vi "DAQX mod 1SDI v02.vi"(0 "resource names":T3={"resource 1"="PXI1Slot2", "resource 2"="PXI1Slot2"}, 1 "close (T)":bool=TRUE, 2 "Record Data":bool, 3 "numSamples":i32=-1, 4 "max time (s)":dbl=10.0 caption="max time", 5 "min sample rate":dbl=100000000.0, 6 "File location":path, 7 "error in":errorcluster, 8 "reference position":dbl=50.0, 9 "Additional text":string, 10 "Type of measurement":T4, 11 "Name root":string, 12 "Monitor On":bool, 13 "channel parameters":T6(array[cluster])=[{"channel name"="0", "input impedance"=0, "maximum input frequency"=30000000.0, "vertical coupling"=1, "probe attenuation"=1.0, "vertical range"=2.0, "vertical offset"=0.0, "channel enabled"=TRUE}, {"channel name"="1", "input impedance"=0, "maximum input frequency"=30000000.0, "vertical coupling"=1, "probe attenuation"=1.0, "vertical range"=2.0, "vertical offset"=0.0, "channel enabled"=TRUE}] {"input impedance" items=["1 mega ohm"=0, "50 ohms"=2]; "vertical coupling" items=["AC", "DC", "Ground"]}, 15 "reset sn":bool) -> (16 "wfm out 1":waveform(dbl)[](array[waveform]), 18 "wfm out 2":waveform(dbl)[](array[waveform]), 19 "file saved":path, 22 "Parameters values file":string, 24 "actualSamples 2":i32, 26 "actualSamples 3":i32, 27 "error out 2":errorcluster caption="error out final")   [LabVIEW 2013]
doc: "Configures and acquires data from an NI-SCOPE high-speed digitizer.\n--------------------\n\nThis Express VI is configured as follows:\n\nDevice: PXI1Slot2 (PXI-5122)\nSample Rate (S/s): 100M\nRecord length: 2k\nAcquisition Mode: N Samples\nChannel 0\n - Range (V): 2\n - Offset (V): 0\n - Probe attenuation: 1\n - Coupling: \n - Input impedence: 1 \n - Bandwidth (Hz): 0\nChannel 1\n - Range (V): 2\n - Offset (V): 0\n - Probe attenuation: 1\n - Coupling: \n - Input impedence: 1 \n - Bandwidth (Hz): 0\nImmediate"
uses:
  <instrlib>/niScope/Controls/niScope vertical coupling.ctl
  Strict Type Defs/type_meas_enum.ctl
  <instrlib>/niScope/Controls/niScope timestamp type.ctl
  <instrlib>/niScope/Controls/niScope clock sync pulse source.ctl
  <instrlib>/niScope/Controls/niScope trigger source digital.ctl
  <instrlib>/niScope/Controls/niScope export destinations.ctl
  <instrlib>/niScope/Controls/niScope exportable signals.ctl
  <instrlib>/niScope/Acquire/Fetch/niScope Multi Fetch Binary 16.vi
  <instrlib>/niScope/Configure/Trigger/niScope Configure Trigger Digital.vi
  <instrlib>/niScope/Configure/Trigger/niScope Configure Trigger Immediate.vi
  shotnoise.vi
  <instrlib>/niScope/Acquire/Fetch/niScope Multi Fetch WDT.vi
panel:
  out "error out 1":errorcluster caption="error out final"
  out "actualSamples 1":i32
  out "actualSamples 0":i32
  out "Chan 1 params":T1
  out "Chan 0 params":T1
  out "actual sample rate":T2
  out "Chan 3 params":T1
  out "Chan 2 params":T1
  out "file location into parameter files":path
  out "size(s)":i32
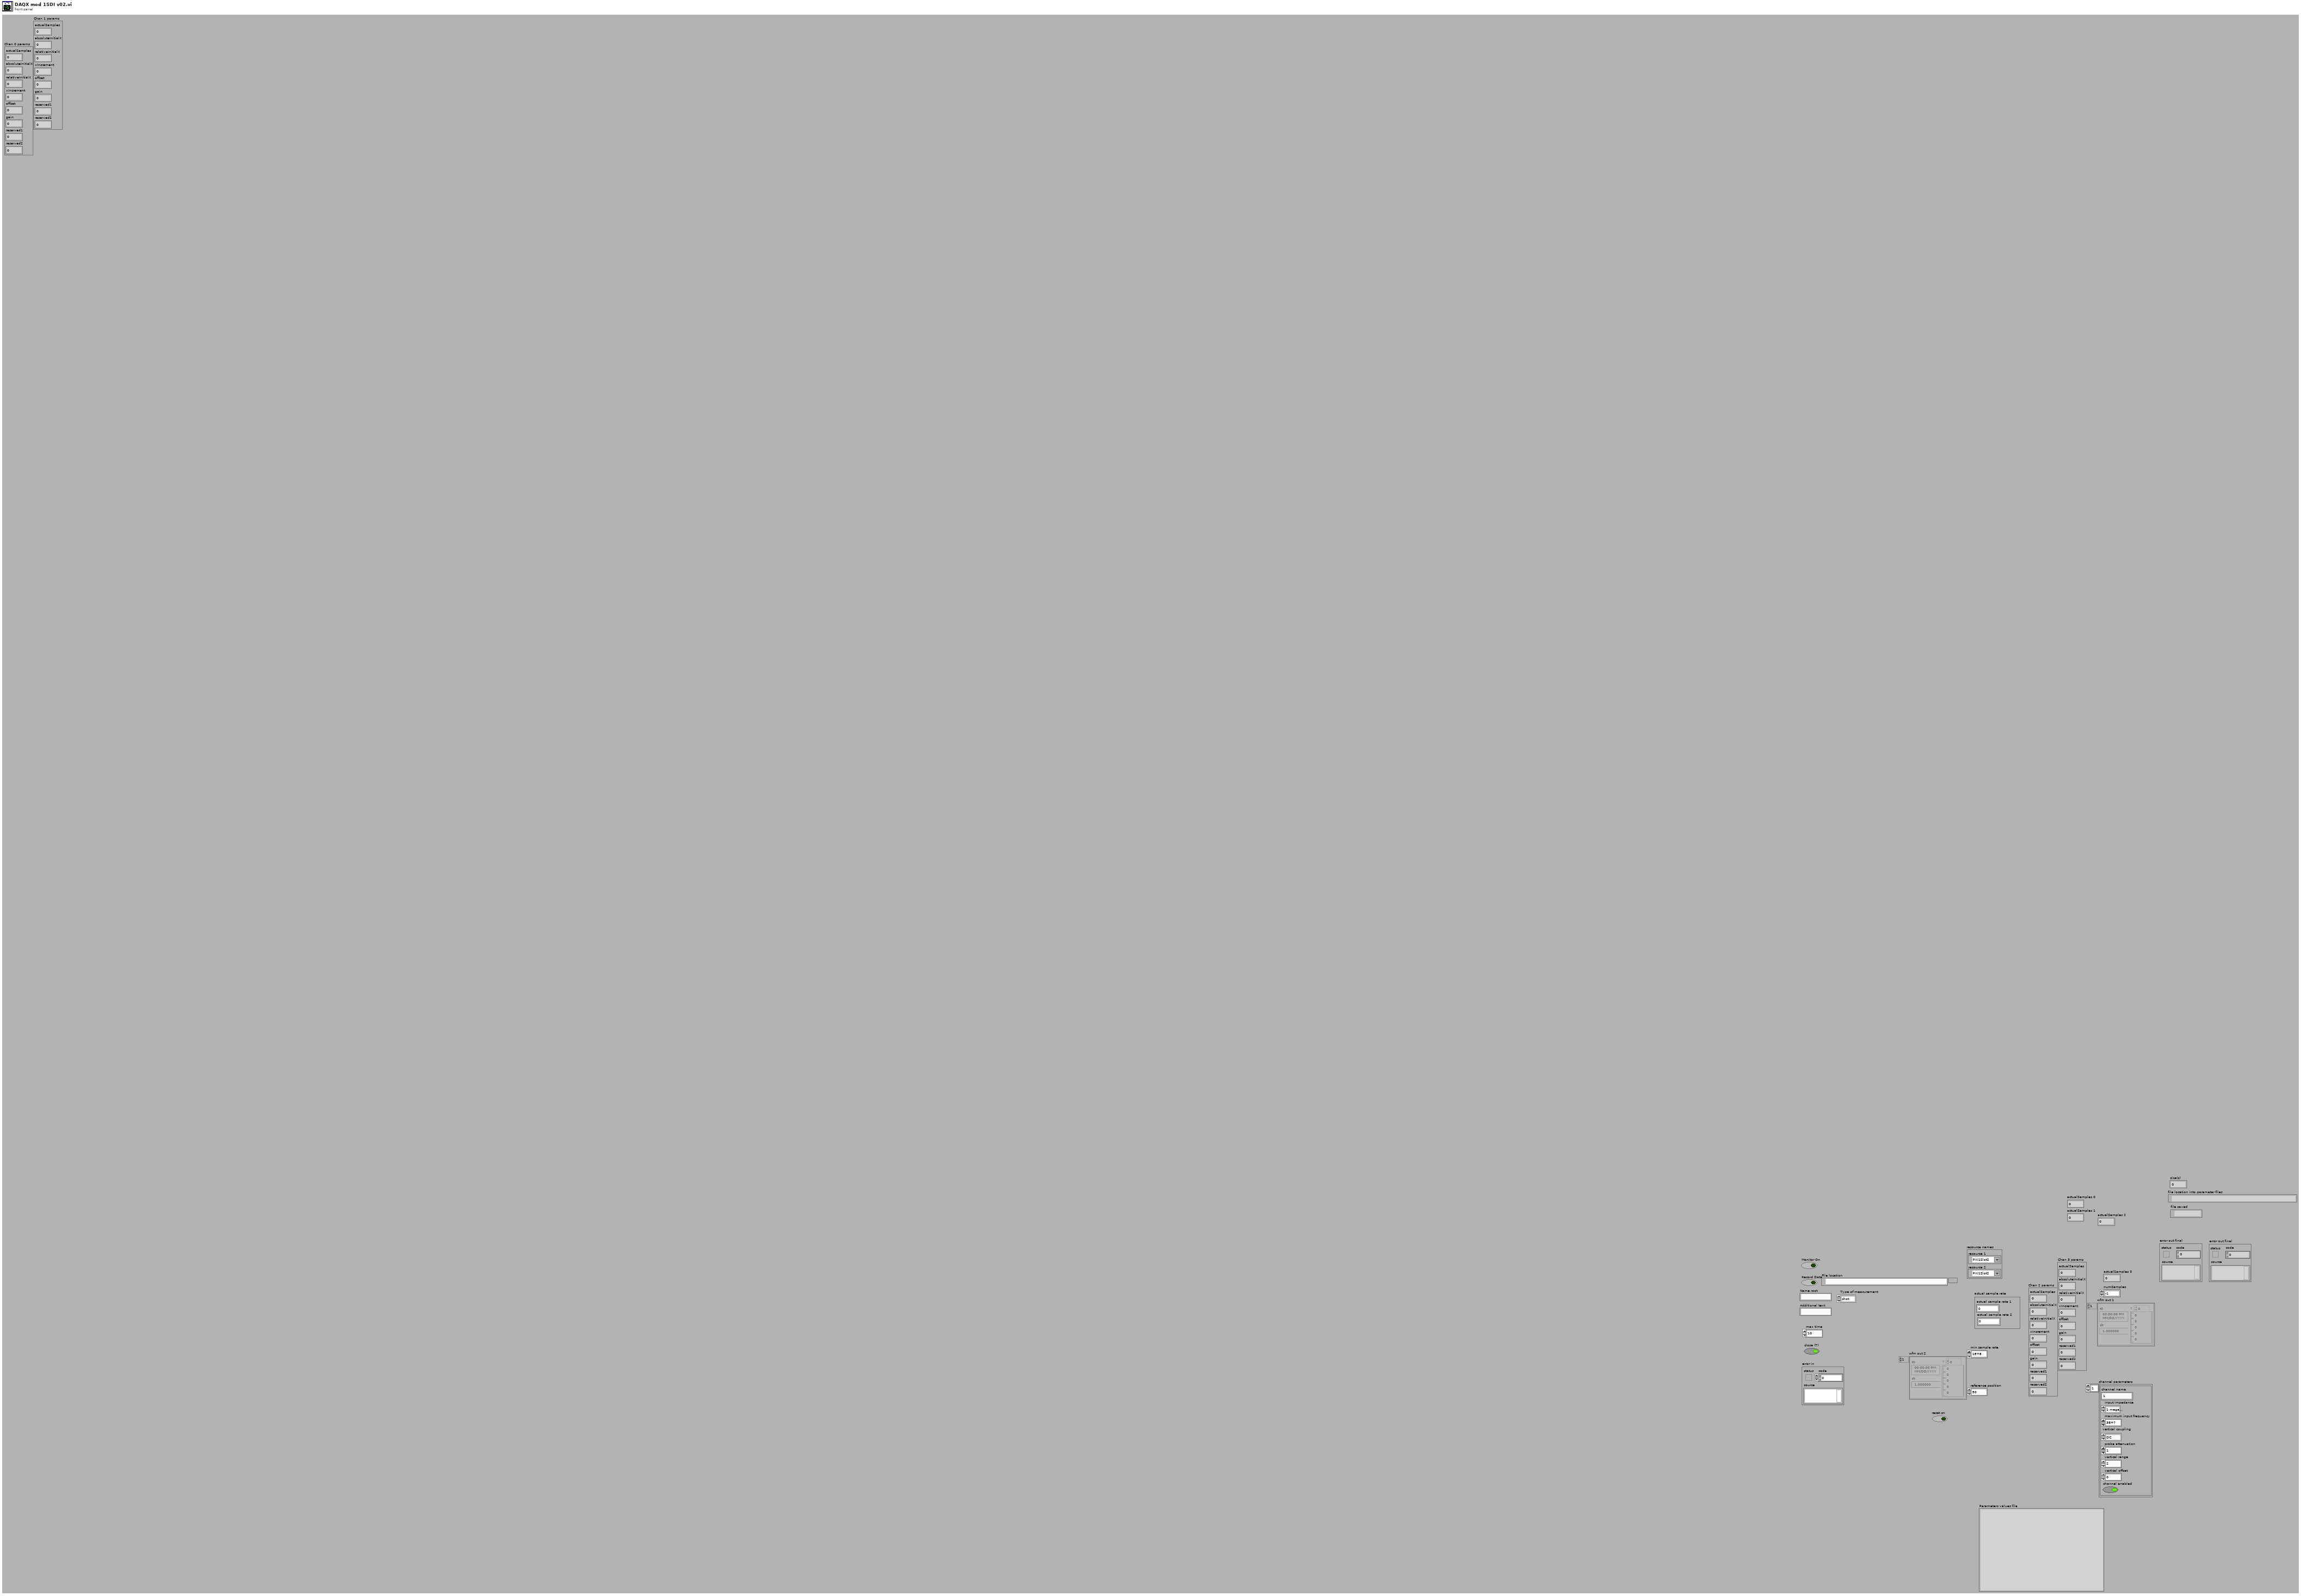
[diagram p1: front panel]
types:
  T1 = cluster{"actualSamples":i32, "absoluteInitialX":dbl, "relativeInitialX":dbl, "xIncrement":dbl, "offset":dbl, "gain":dbl, "reserved1":dbl, "reserved2":dbl}
  T2 = cluster{"actual sample rate":dbl, "actual sample rate 2":dbl}
  T3 = cluster{"resource 1":refnum<k15>, "resource 2":refnum<k15>}
  T4 = typedef "type_meas_enum.ctl" = enum16{"shot", "x", "p", "electronic"}
  T5 = typedef "niScope vertical coupling.ctl" = i32
  T6 = cluster{"channel name":string, "input impedance":u32, "maximum input frequency":dbl, "vertical coupling":T5, "probe attenuation":dbl, "vertical range":dbl, "vertical offset":dbl, "channel enabled":bool}[]
  T7 = typedef "niScope timestamp type.ctl" = i32
  T8 = typedef "niScope export destinations.ctl" = string
  T9 = typedef "niScope trigger source digital.ctl" = string
  T10 = typedef "niScope exportable signals.ctl" = u16
  T11 = typedef "niScope clock sync pulse source.ctl" = u16
  T12 = cluster{"actual sample rate":dbl, "actual sample rate":dbl}
  T13 = cluster{"actualSamples":i32, "absoluteInitialX":dbl, "relativeInitialX":dbl, "xIncrement":dbl, "offset":dbl, "gain":dbl, "reserved1":dbl, "reserved2":dbl}[]
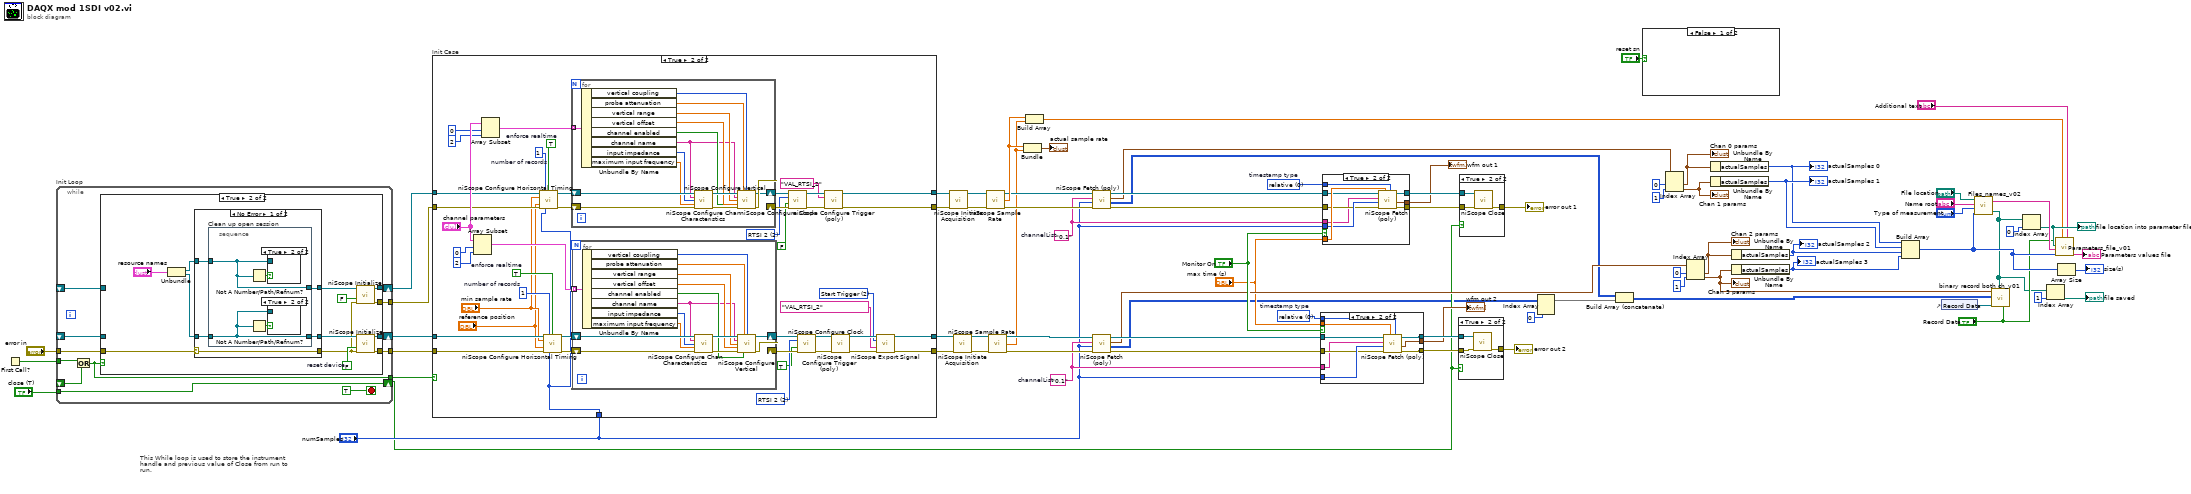
[diagram p0: block diagram]
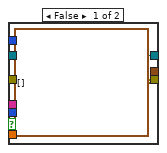
[diagram p3: hidden frame]
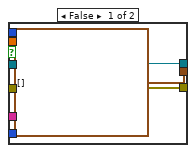
[diagram p4: hidden frame]
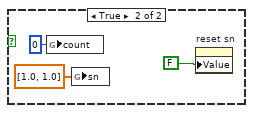
[diagram p5: hidden frame]
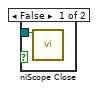
[diagram p7: hidden frame]
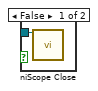
[diagram p8: hidden frame]
diagram:
  w28 = T7 0 items=["relative", "absolute"]  # timestamp type
  w31 = "0,1"  # channelList
  w44 = "0,1"  # channelList
  w78 = T7 0 items=["relative", "absolute"]  # timestamp type
  # "This While loop is used to store the instrument handle and previous value of Close from run to run."
  n1 = First Call?() -> (First Call?: T/F=w77:bool)
  n2 = while "Init Loop" {
    tunnel: w77 -> [w91]
    shift-right: [w90] -> w22
    shift-left: _ -> [w87]
    tunnel: "close (T)" -> [w90]
    shift-right: [w89] -> w76
    shift-left: _ -> [w88]
    tunnel: [w85] -> w75
    tunnel: "error in" -> [w84]
    tunnel: [w80] -> w74
    shift-right: [w83] -> w39
    shift-left: _ -> [w82]
    tunnel: [w81] -> w40
    stop <- TRUE ("stopInit") stop-if-true
    n3 = Or(x=w91, y=w87) -> (x .or. y?=w80:bool)
    n4 = case "Select_Init" shown="True" w80 {
      tunnel: [w94 w105] -> w89
      tunnel: w88 -> [w94 _]
      tunnel: [w92 w104] -> w85
      tunnel: w84 -> [w92 w103]
      tunnel: [w93 w98] -> w83
      tunnel: w82 -> [w93 _]
      tunnel: [w92 w95] -> w81
      frame False {
      }
      frame True {
        w106 = FALSE  # reset device
        n5 = Unbundle("resource names") -> ("resource 1"=w100:refnum<k15>, "resource 2"=w101:refnum<k15>)
        n6 = case shown="No Error" w103 {
          selector: w103 -> [w110 w120]
          tunnel: [w112 w121] -> w107
          tunnel: w101 -> [w111 w121]
          tunnel: [w110 w120] -> w97
          tunnel: w100 -> [w109 w119]
          tunnel: [w108 w119] -> w99
          frame No Error {
            n7 = stacked-sequence "Clean up open session" {
              tunnel: w111 -> [w115]
              tunnel: [w115] -> w112
              tunnel: w109 -> [w113]
              tunnel: [w113] -> w108
              frame #0 {
                n8 = Not A Number/Path/Refnum?(number/path/refnum=w113) -> (NaN/Path/Refnum?=w114:bool)
                n9 = Not A Number/Path/Refnum?(number/path/refnum=w115) -> (NaN/Path/Refnum?=w116:bool)
                n10 = case shown="True" w114 {
                  tunnel: w113 -> [w117 _]
                  frame False {
                    n11 = call <instrlib>:"niScope Close.vi"("instrument handle"=w117) -> ()  [unwired: 1 in, 14 out]
                  }
                  frame True {
                  }
                }
                n12 = case shown="True" w116 {
                  tunnel: w115 -> [w118 _]
                  frame False {
                    n13 = call <instrlib>:"niScope Close.vi"("instrument handle"=w118) -> ()  [unwired: 1 in, 14 out]
                  }
                  frame True {
                  }
                }
              }
            }
          }
          frame Error {
          }
        }
        n14 = call <instrlib>:"niScope Initialize.vi"("resource name"=w99, "reset device"=FALSE, "error in"=w97) -> ("instrument handle"=w98:refnum<k15>, "error out"=w95:errorcluster)  [unwired: 2 in, 9 out]
        n15 = call <instrlib>:"niScope Initialize.vi"("resource name"=w107, "reset device"=w106, "error in"=w97) -> ("instrument handle"=w105:refnum<k15>, "error out"=w104:errorcluster)  [unwired: 2 in, 9 out]
      }
    }
  }
  n16 = case "Init Case" shown="True" w74 {
    tunnel: w75 -> [w124 w163]
    tunnel: [w124 w132] -> w7
    tunnel: [w125 w133] -> w8
    tunnel: w76 -> [w125 w164]
    tunnel: "numSamples" -> [_ w128]
    tunnel: w40 -> [w122 w153]
    tunnel: w39 -> [w123 w152]
    tunnel: [w123 w127] -> w6
    tunnel: [w122 w126] -> w5
    frame False {
    }
    frame True {
      w131 = T10 2 items=["None"=0, "Start Trigger"=2, "Advance Trigger"=5, "Reference Trigger"=1, "End of Record Event"=4, "End of Acquisition Event"=3, "Ready for Start Event"=7, "Ready for Advance Event"=6, "Ready for Reference Event"=10, "Reference Clock"=100, "Sample Clock"=101, "5 Volt Power"=13] ("signal")
      w144 = T11 2 items=["RTSI 0", "RTSI 1", "RTSI 2", "RTSI 3", "RTSI 4", "RTSI 5", "RTSI 6", "PFI 1", "PFI 2", "Internal"] ("clock sync pulse source")
      w145 = T11 2 items=["RTSI 0", "RTSI 1", "RTSI 2", "RTSI 3", "RTSI 4", "RTSI 5", "RTSI 6", "PFI 1", "PFI 2", "Internal"] ("clock sync pulse source")
      w151 = 1  # number of records
      w150 = TRUE  # enforce realtime
      w167 = 1  # number of records
      w168 = TRUE  # enforce realtime
      n17 = Array Subset(array="channel parameters", index=0, length=2) -> (w160:T6)
      n18 = Array Subset(array="channel parameters", index=0, length=2) -> (w158:T6)
      n19 = call <instrlib>:"niScope Configure Horizontal Timing.vi"("instrument handle"=w152, "number of records"=w151, "enforce realtime"=w150, "min sample rate"="min sample rate", "reference position"="reference position", "error in"=w153, "min record length"=w128) -> ("instrument handle out"=w155:refnum<k15>, "error out"=w154:errorcluster)  [unwired: 7 out]
      n20 = call <instrlib>:"niScope Configure Horizontal Timing.vi"("instrument handle"=w164, "number of records"=w167, "enforce realtime"=w168, "min sample rate"="min sample rate", "reference position"="reference position", "error in"=w163, "min record length"=w128) -> ("instrument handle out"=w165:refnum<k15>, "error out"=w166:errorcluster)  [unwired: 7 out]
      n21 = for {
        shift-right: [w171] -> w148
        shift-left: w154 -> [w183]
        shift-right: [w170] -> w149
        shift-left: w155 -> [w182]
        tunnel: w158 -> [w179] mode=indexing
        n22 = Unbundle By Name(w179) -> ("vertical coupling"=w176:T5, "probe attenuation"=w175:dbl, "vertical range"=w174:dbl, "vertical offset"=w173:dbl, "channel enabled"=w172:bool, "channel name"=w169:string, "input impedance"=w177:u32, "maximum input frequency"=w178:dbl)
        n23 = call <instrlib>:"niScope Configure Chan Characteristics.vi"("instrument handle"=w182, "channels"=w169, "input impedance"=w177, "maximum input frequency"=w178, "error in"=w183) -> ("instrument handle out"=w181:refnum<k15>, "error out"=w180:errorcluster)  [unwired: 9 out]
        n24 = call <instrlib>:"niScope Configure Vertical.vi"("instrument handle"=w181, "probe attenuation"=w175, "vertical coupling"=w176, "channels"=w169, "vertical range"=w174, "vertical offset"=w173, "error in"=w180, "channel enabled"=w172) -> ("instrument handle out"=w170:refnum<k15>, "error out"=w171:errorcluster)  [unwired: 6 out]
      }
      n25 = for {
        shift-right: [w186] -> w146
        shift-left: w166 -> [w198]
        shift-right: [w185] -> w147
        shift-left: w165 -> [w197]
        tunnel: w160 -> [w194] mode=indexing
        n26 = Unbundle By Name(w194) -> ("vertical coupling"=w191:T5, "probe attenuation"=w190:dbl, "vertical range"=w189:dbl, "vertical offset"=w188:dbl, "channel enabled"=w187:bool, "channel name"=w184:string, "input impedance"=w192:u32, "maximum input frequency"=w193:dbl)
        n27 = call <instrlib>:"niScope Configure Chan Characteristics.vi"("instrument handle"=w197, "channels"=w184, "input impedance"=w192, "maximum input frequency"=w193, "error in"=w198) -> ("instrument handle out"=w196:refnum<k15>, "error out"=w195:errorcluster)  [unwired: 9 out]
        n28 = call <instrlib>:"niScope Configure Vertical.vi"("instrument handle"=w196, "probe attenuation"=w190, "vertical coupling"=w191, "channels"=w184, "vertical range"=w189, "vertical offset"=w188, "error in"=w195, "channel enabled"=w187) -> ("instrument handle out"=w185:refnum<k15>, "error out"=w186:errorcluster)  [unwired: 6 out]
      }
      n29 = call <instrlib>:"niScope Configure Clock.vi"("instrument handle"=w149, "clock sync pulse source"=w144, "master enabled"=FALSE, "error in"=w148) -> ("instrument handle out"=w136:refnum<k15>, "error out"=w137:errorcluster)  [unwired: 10 in]
      n30 = call <instrlib>:"niScope Configure Clock.vi"("instrument handle"=w147, "clock sync pulse source"=w145, "master enabled"=TRUE, "error in"=w146) -> ("instrument handle out"=w141:refnum<k15>, "error out"=w140:errorcluster)  [unwired: 10 in]
      n31 = call-poly <instrlib>:"niScope Configure Trigger (poly).vi"("instrument handle"=w136, "trigger source"=T9 "VAL_RTSI_2", "error in"=w137) -> ("instrument handle out"=w127:refnum<k15>, "error out"=w126:errorcluster)  [unwired: 3 in, 8 out]
      n32 = call-poly <instrlib>:"niScope Configure Trigger (poly).vi"("instrument handle"=w141, "error in"=w140) -> ("instrument handle out"=w139:refnum<k15>, "error out"=w138:errorcluster)  [unwired: 12 out]
      n33 = call <instrlib>:"niScope Export Signal.vi"("instrument handle"=w139, "signal"=w131, "output terminal"=T8 "VAL_RTSI_2", "error in"=w138) -> ("instrument handle out"=w133:refnum<k15>, "error out"=w132:errorcluster)  [unwired: 10 in]
    }
  }
  n34 = call <instrlib>:"niScope Initiate Acquisition.vi"("instrument handle"=w6, "error in"=w5) -> ("instrument handle out"=w2:refnum<k15>, "error out"=w1:errorcluster)  [unwired: 12 out]
  n35 = call <instrlib>:"niScope Initiate Acquisition.vi"("instrument handle"=w8, "error in"=w7) -> ("instrument handle out"=w4:refnum<k15>, "error out"=w3:errorcluster)  [unwired: 12 out]
  n36 = call <instrlib>:"niScope Sample Rate.vi"("instrument handle"=w2, "error in"=w1) -> ("instrument handle out"=w36:refnum<k15>, "actual sample rate"=w37:dbl, "error out"=w35:errorcluster)  [unwired: 11 out]
  n37 = call <instrlib>:"niScope Sample Rate.vi"("instrument handle"=w4, "error in"=w3) -> ("instrument handle out"=w69:refnum<k15>, "actual sample rate"=w32:dbl, "error out"=w68:errorcluster)  [unwired: 11 out]
  n38 = Bundle("actual sample rate"=w37, "actual sample rate"=w32) -> (→"actual sample rate":T12)  [unwired: 1 in]
  n39 = Build Array(w37, w32) -> (w56:dbl[])
  n40 = call-poly <instrlib>:"niScope Fetch (poly).vi"("error in"=w35, "numSamples"="numSamples", "channels"=w31, "instrument handle"=w36) -> ("error out"=w33:errorcluster, "wfm"=w16:i16[][], "wfm info"=w17:T13, "instrument handle out"=w34:refnum<k15>)  [unwired: 1 in, 3 out]
  n41 = call-poly <instrlib>:"niScope Fetch (poly).vi"("error in"=w68, "numSamples"="numSamples", "channels"=w44, "instrument handle"=w69) -> ("error out"=w52:errorcluster, "wfm"=w13:i16[][], "wfm info"=w27:T13, "instrument handle out"=w53:refnum<k15>)  [unwired: 1 in, 3 out]
  n42 = case shown="True" "Monitor On" {
    tunnel: "max time (s)" -> [_ w210]
    tunnel: w78 -> [_ w209]
    tunnel: [w200 w208] -> w71
    tunnel: "numSamples" -> [_ w207]
    tunnel: w53 -> [w200 w206]
    tunnel: w52 -> [w201 w205]
    tunnel: [w201 w204] -> w50
    tunnel: [waveform(dbl)[] [] ("wfm") w203] -> w49
    tunnel: w44 -> [_ w202]
    frame False {
    }
    frame True {
      n43 = call-poly <instrlib>:"niScope Fetch (poly).vi"("timestamp Type"=w209, "timeout"=w210, "error in"=w205, "numSamples"=w207, "channels"=w202, "instrument handle"=w206) -> ("error out"=w204:errorcluster, "wfm"=w203:waveform(dbl)[], "instrument handle out"=w208:refnum<k15>)  [unwired: 3 out]
    }
  }
  "wfm out 2" <- w49
  n44 = case shown="True" "Monitor On" {
    tunnel: "max time (s)" -> [_ w222]
    tunnel: w28 -> [_ w221]
    tunnel: [w212 w220] -> w24
    tunnel: "numSamples" -> [_ w219]
    tunnel: w34 -> [w212 w218]
    tunnel: w33 -> [w213 w217]
    tunnel: [w213 w216] -> w25
    tunnel: [waveform(dbl)[] [] ("wfm") w215] -> w23
    tunnel: w31 -> [_ w214]
    frame False {
    }
    frame True {
      n45 = call-poly <instrlib>:"niScope Fetch (poly).vi"("timestamp Type"=w221, "timeout"=w222, "error in"=w217, "numSamples"=w219, "channels"=w214, "instrument handle"=w218) -> ("error out"=w216:errorcluster, "wfm"=w215:waveform(dbl)[], "instrument handle out"=w220:refnum<k15>)  [unwired: 3 out]
    }
  }
  "wfm out 1" <- w23
  n46 = case shown="True" w22 {
    tunnel: w50 -> [w223 w226]
    tunnel: [w223 w225] -> w79
    tunnel: w71 -> [_ w224]
    frame False {
    }
    frame True {
      n47 = call <instrlib>:"niScope Close.vi"("instrument handle"=w224, "error in"=w226) -> ("error out"=w225:errorcluster)  [unwired: 13 out]
    }
  }
  "error out 2" <- w79
  n48 = case shown="True" w22 {
    tunnel: w25 -> [w227 w230]
    tunnel: [w227 w229] -> w9
    tunnel: w24 -> [_ w228]
    frame False {
    }
    frame True {
      n49 = call <instrlib>:"niScope Close.vi"("instrument handle"=w228, "error in"=w230) -> ("error out"=w229:errorcluster)  [unwired: 13 out]
    }
  }
  "error out 1" <- w9
  n50 = Index Array(array=w13, index (col)=0 ("index (row)")) -> (element=w11:i16[])  [unwired: 1 in]
  n51 = Build Array (concatenate)(w16, w11) -> (w12:i16[][])
  n52 = case shown="False" "reset sn" {
    frame False {
    }
    frame True {
      n53 = global write "shotnoise.vi" "count"(i64 0 ("count")) -> ()
      n54 = global write "shotnoise.vi" "sn"(dbl[] [1.0, 1.0] ("sn")) -> ()
      n55 = property on="reset sn" class="Bool (strict)"("Value"=FALSE ("reset sn")) -> ()  [unwired: 2 in, 2 out]
    }
  }
  n56 = Index Array(array=w17, index #1=0 ("index"), index #2=1 ("index")) -> (element #1=w19:T1, element #2=w18:T1)
  "Chan 0 params" <- w19
  "Chan 1 params" <- w18
  n57 = Index Array(array=w27, index #1=0 ("index"), index #2=1 ("index")) -> (element #1=w65:T1, element #2=w46:T1)
  "Chan 2 params" <- w65
  "Chan 3 params" <- w46
  n58 = Unbundle By Name(w19) -> ("actualSamples"=w14:i32)
  "actualSamples 0" <- w14
  n59 = Unbundle By Name(w18) -> ("actualSamples"=w15:i32)
  "actualSamples 1" <- w15
  n60 = Unbundle By Name(w65) -> ("actualSamples"=w64:i32)
  "actualSamples 2" <- w64
  n61 = Unbundle By Name(w46) -> ("actualSamples"=w48:i32)
  "actualSamples 3" <- w48
  n62 = Build Array(w14, w15, w64, w48) -> (w55:i32[])
  n63 = control-ref of="Record Data"() -> (w47:refnum<vi>)
  n64 = call "Files_names_v02.vi"("actualSamples\narray"=w55, "Type of\nmeasurement"="Type of measurement", "Name root"="Name root", "File location"="File location") -> ("Files path array"=w43:path[], "Files name array"=w60:string[])
  n65 = call "binary record both ch_v01.vi"("Record"="Record Data", "Files path array"=w43, "reference"=w47, "wfm"=w12, "Chan 1 params"=w46) -> ()  [unwired: 7 in]
  n66 = Index Array(array=w43, index=0) -> (element=w58:path)
  "file location into parameter files" <- w58
  n67 = Index Array(array=w43, index=1) -> (element=→"file saved":path)
  n68 = call "Parameters_file_v01.vi"("Additional text"="Additional text", "actual sample rate array"=w56, "actualSamples array"=w55, "Files name array"=w60, "File location"=w58, "Record"="Record Data") -> ("Full text"=→"Parameters values file":string)  [unwired: 3 in]
  n69 = Array Size(array=w55) -> (size(s)=→"size(s)":i32)
